vi "CSTK_Icon_Creator_Dialong_InputPath.vi"(0 "Enable":bool=TRUE caption="启用", 1 "分类文件夹名输入":string caption="分类文件夹名", 5 "error in (no error)":errorcluster caption="错误输入（无错误）") -> (17 "分类文件夹名输出":string caption="分类文件夹名", 18 "确定":bool, 19 "error out":errorcluster caption="错误输出")   [LabVIEW 2015, in "CSTK_Icon Creator.lvlib"]
doc: "显示标准对话框，提示用户输入用户名、密码等信息。\n--------------------\n\n该Express VI配置如下:\n\n显示给用户的信息:请输入分类文件夹名\n该输入为: \n文本输入框: 分类文件夹名"
uses:
  CSTK_Icon Creator.lvlib
panel:
  in  "分类文件夹名":string
  in  "Cancel":bool caption="取消"
  in  "OK2":bool
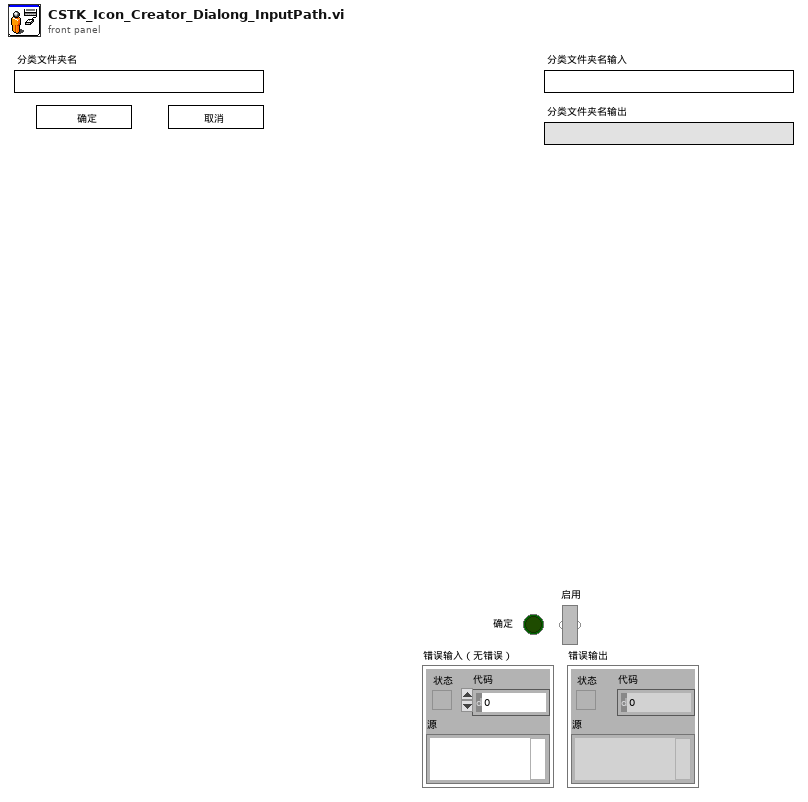
[diagram p1: front panel]
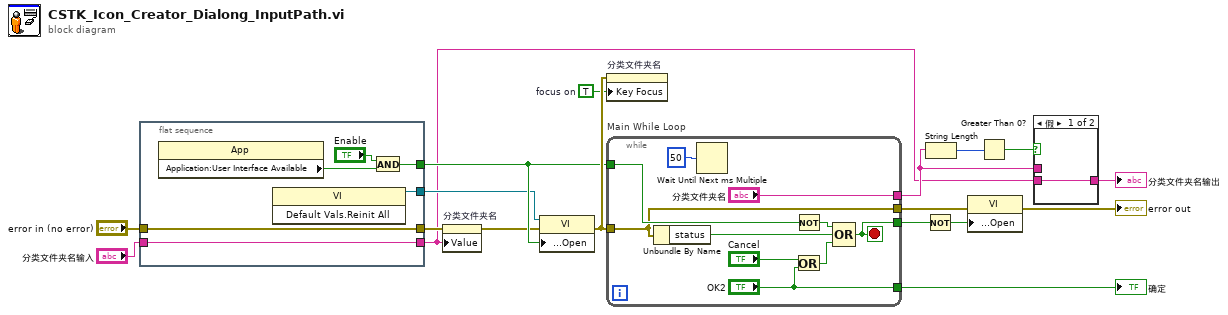
[diagram p0: block diagram]
diagram:
  w11 = TRUE  # focus on
  n1 = flat-sequence {
    tunnel: [w23] -> w13
    tunnel: [w21] -> w12
    tunnel: [w20] -> w8
    tunnel: "error in (no error)" -> [w20]
    tunnel: [w19] -> w1
    tunnel: "分类文件夹名输入" -> [w19]
    frame #0 {
      n2 = property class="App"() -> ("Application:User Interface Available"=w22:bool)  [unwired: 2 in, 2 out]
      n3 = invoke class="VI" method="Default Vals.Reinit All"() -> (reference out=w21:refnum<vi>)  [unwired: 3 in, 2 out]
      n4 = And(x="Enable", y=w22) -> (x .and. y?=w23:bool)
    }
  }
  n5 = property on="分类文件夹名" class="Str"(error in=w8, "Value"=w1) -> (error out=w7:errorcluster)  [unwired: 1 in, 1 out]
  n6 = property class="VI"(reference=w12, error in=w7, "Front Panel Window:Open"=w13) -> (error out=w16:errorcluster)  [unwired: 1 out]
  n7 = property on="分类文件夹名" class="Str"(error in=w16, "Key Focus"=w11) -> ()  [unwired: 1 in, 2 out]
  n8 = while "Main While Loop" {
    tunnel: ["OK2"] -> w6
    tunnel: w13 -> [w32]
    tunnel: [w30] -> w17
    tunnel: w16 -> [w29]
    tunnel: [w29] -> w15
    tunnel: ["分类文件夹名"] -> w2
    stop <- w30 stop-if-true
    n9 = Unbundle By Name(w29) -> ("status"=w27:bool)
    n10 = Wait Until Next ms Multiple(millisecond multiple=u32 50) -> ()  [unwired: 1 out]
    n11 = Not(x=w32) -> (.not. x?=w31:bool)
    n12 = Or(x="Cancel", y="OK2") -> (x .or. y?=w28:bool)
    n13 = Compound Arithmetic op=OR(w31, w27, w28) -> (w30:bool)
  }
  "确定" <- w6
  n14 = Not(x=w17) -> (.not. x?=w18:bool)
  n15 = String Length(string=w2) -> (length=w5:i32)
  n16 = property class="VI"(error in=w15, "Front Panel Window:Open"=w18) -> (error out=→"error out":errorcluster)  [unwired: 1 in, 1 out]
  n17 = Greater Than 0?(x=w5) -> (x > 0?=w4:bool)
  n18 = case shown="假" w4 {
    tunnel: [w35 w36] -> w3
    tunnel: w2 -> [_ w36]
    tunnel: w1 -> [w35 _]
    frame False {
    }
    frame True {
    }
  }
  "分类文件夹名输出" <- w3
